vi "CRC.vi"(1 "Packet byte array":u8[](array[numeric])) -> (0 "CRC Error":bool)   [LabVIEW 2015]
panel:
  out "CRC":u8
  out "calcCRC":u8
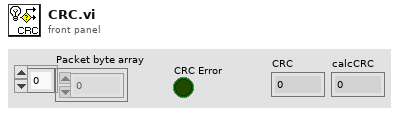
[diagram p1: front panel]
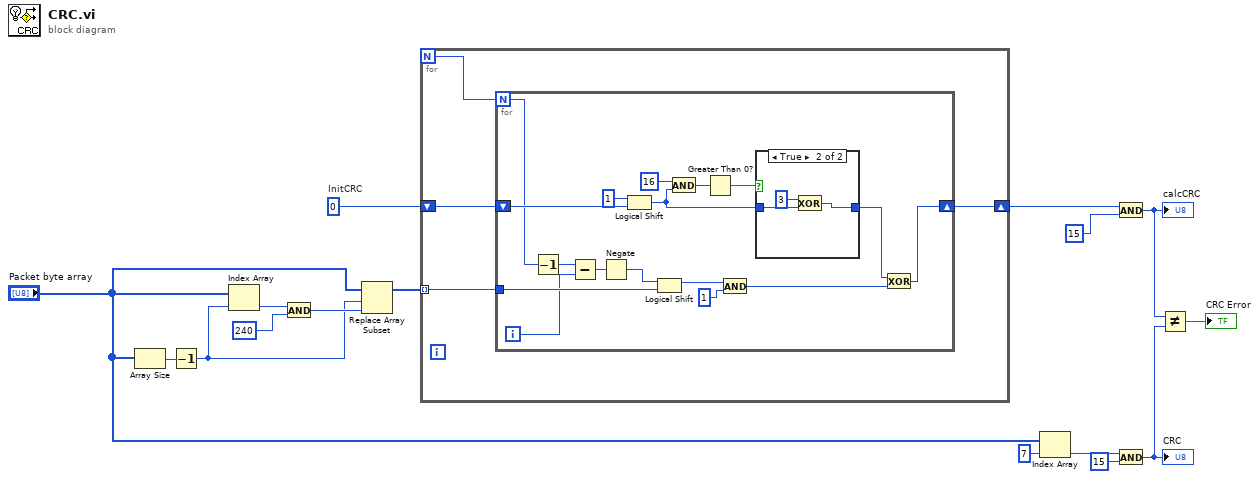
[diagram p0: block diagram]
diagram:
  w16 = u8 0  # InitCRC
  n1 = Array Size(array="Packet byte array") -> (size(s)=w6:i32)
  n2 = Decrement(x=w6) -> (x-1=w5:i32)
  n3 = Index Array(array="Packet byte array", index=w5) -> (element=w10:u8)
  n4 = And(x=w10, y=u8 240) -> (x .and. y?=w8:u8)
  n5 = Replace Array Subset(array="Packet byte array", new element=w8, index=w5) -> (w7:u8[])
  n6 = for {
    N -> [w17]
    tunnel: w7 -> [w19] mode=indexing
    shift-right: [w18] -> w15
    shift-left: w16 -> [w20]
    n7 = for {
      N: w17 -> [w21]
      tunnel: w19 -> [w31]
      shift-right: [w26] -> w18
      shift-left: w20 -> [w33]
      i -> [w30]
      n8 = Decrement(x=w21) -> (x-1=w22:i32)
      n9 = Subtract(x=w22, y=w30) -> (x-y=w29:i32)
      n10 = Negate(x=w29) -> (-x=w23:i32)
      n11 = Logical Shift(y=u8 1 ("x"), x=w33) -> (x << y=w34:u8)
      n12 = Logical Shift(y=w23, x=w31) -> (x << y=w28:u8)
      n13 = And(x=u8 16, y=w34) -> (x .and. y?=w36:u8)
      n14 = Greater Than 0?(x=w36) -> (x > 0?=w35:bool)
      n15 = And(x=w28, y=u8 1) -> (x .and. y?=w24:u8)
      n16 = case shown="True" w35 {
        tunnel: w34 -> [w38 w41]
        tunnel: [w38 w39] -> w25
        frame False {
        }
        frame True {
          n17 = Exclusive Or(1:w41, 2:u8 3 ("x")) -> (0:w39:u8)
        }
      }
      n18 = Exclusive Or(1:w24, 2:w25) -> (0:w26:u8)
    }
  }
  n19 = Index Array(array="Packet byte array", index=7) -> (element=w12:u8)
  n20 = And(x=w15, y=u8 15) -> (x .and. y?=w4:u8)
  "calcCRC" <- w4
  n21 = And(x=w12, y=u8 15) -> (x .and. y?=w3:u8)
  "CRC" <- w3
  n22 = Not Equal?(x=w4, y=w3) -> (x != y?=→"CRC Error":bool)
